vi "Dashboard Main.vi"() -> ()   [LabVIEW 2011]
uses:
  <vilib>/Rock Robotics/WPI/DriverStation/WPI_DriverStationDigitalData.ctl
panel:
  out "8 -- Battery":sgl(graph)
  out "Analog Input":sgl[](array[slide]) scale=0.0..5.0
  in  "Viewer":enum32{"Camera Image", "Kinect Skeleton"}(tab)
  in  "Video Enable":bool=TRUE
  out "Camera Image":T1(plugin-control)
  out "Buttons 1":cluster{"1":bool, "2":bool, "3":bool}
  out "Kinect 1":cluster{"X":dbl, "Y":dbl, "Z":dbl} {"X" scale=1.0..-1.0; "Y" scale=1.0..-1.0; "Z" scale=1.0..-1.0}
  out "Buttons 2":cluster{"1":bool, "2":bool, "3":bool}
  out "Kinect 2":cluster{"X":dbl, "Y":dbl, "Z":dbl} {"X" scale=1.0..-1.0; "Y" scale=1.0..-1.0; "Z" scale=1.0..-1.0}
  out "Version":string
  out "Skeleton Picture":picture
  out "Players":i8
  out "Dashboard Datatype Warning":string="Warning: The Dashboard Datatype used by the robot project and this dashboard do not match.\nSee diagram for more details."
  out "Robot IP Address":string
  out "Image Error Message":string="Timeout in Camera Communications"
  out "Solenoid Output":bool[](array[boolean])
  out "PWM":cluster{u8, u8}[](array[slide])=[{0, 157}, {0, 157}, {0, 157}, {0, 157}, {0, 157}, {0, 157}, {0, 157}, {0, 157}, {0, 157}, {0, 169}] scale=1.0..255.0
  out "GPIO Output Enable":bool[](array[boolean])
  out "GPIO State":bool[](array[boolean])
  out "Relay":cluster{"Forward":bool[], "Reverse":bool[]}
  # "Analog #1"
  # "1"
  # "7"
  # "Communications"
  # "Solenoid #1"
  # "1"
  # "8"
  # "Digital #1"
  # "1"
  # "10"
  # "1"
  # "14"
  # "1"
  # "8"
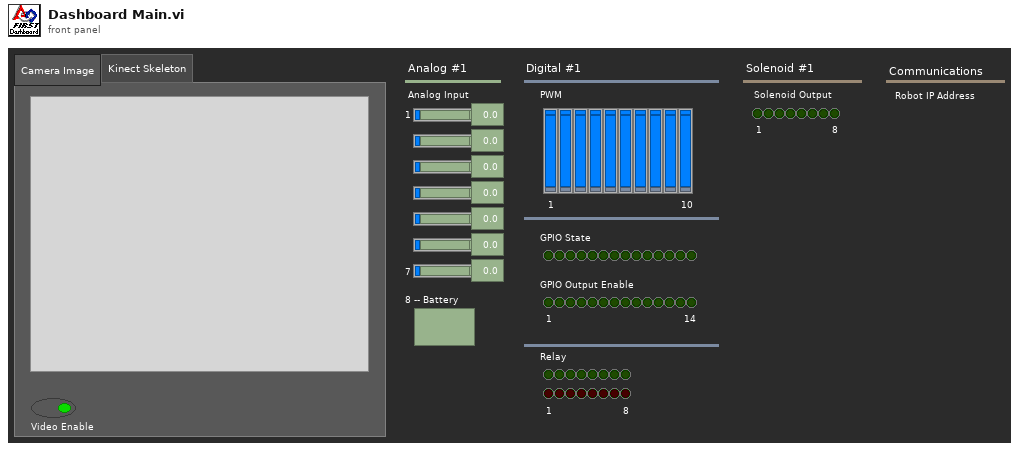
[diagram p1: front panel]
types:
  T1 = typedef "IMAQ Image.ctl" = refnum<image>
  T2 = typedef "WPI_DriverStationDigitalData.ctl" = cluster{"Relay Fwd":u8, "Relay Rev":u8, "GPIO":u16, "GPIO_OE":u16, "PWM":cluster{"PWM[0]":u8, "PWM[1]":u8, "PWM[2]":u8, "PWM[3]":u8, "PWM[4]":u8, "PWM[5]":u8, "PWM[6]":u8, "PWM[7]":u8, "PWM[8]":u8, "PWM[9]":u8}}
  T3 = cluster{cluster{"AnalogModule[0]":cluster{"Channel[0]":sgl, "Channel[1]":sgl, "Channel[2]":sgl, "Channel[3]":sgl, "Channel[4]":sgl, "Channel[5]":sgl, "Channel[6]":sgl, "Channel[7]":sgl}, "AnalogModule[1]":cluster{"Channel[0]":sgl, "Channel[1]":sgl, "Channel[2]":sgl, "Channel[3]":sgl, "Channel[4]":sgl, "Channel[5]":sgl, "Channel[6]":sgl, "Channel[7]":sgl}}, cluster{"DigitalModule[0]":T2, "DigitalModule[1]":T2}, "Solenoid":u8}
  T4 = typedef "Image Type" = u32
  T5 = cluster{"Competition mode":bool, "Robot Link":bool, "Autonomous":bool, "Enabled":bool, "E-Stop":bool}
  T6 = cluster{"AnalogModule[0]":cluster{"Channel[0]":sgl, "Channel[1]":sgl, "Channel[2]":sgl, "Channel[3]":sgl, "Channel[4]":sgl, "Channel[5]":sgl, "Channel[6]":sgl, "Channel[7]":sgl}, "AnalogModule[1]":cluster{"Channel[0]":sgl, "Channel[1]":sgl, "Channel[2]":sgl, "Channel[3]":sgl, "Channel[4]":sgl, "Channel[5]":sgl, "Channel[6]":sgl, "Channel[7]":sgl}}
  T7 = cluster{"DigitalModule[0]":T2, "DigitalModule[1]":T2}
  T8 = cluster{"Channel[0]":sgl, "Channel[1]":sgl, "Channel[2]":sgl, "Channel[3]":sgl, "Channel[4]":sgl, "Channel[5]":sgl, "Channel[6]":sgl, "Channel[7]":sgl}[]
  T9 = cluster{"Channel[0]":sgl, "Channel[1]":sgl, "Channel[2]":sgl, "Channel[3]":sgl, "Channel[4]":sgl, "Channel[5]":sgl, "Channel[6]":sgl, "Channel[7]":sgl}
  T10 = typedef "LVRectTypeDef.ctl" = cluster{"left":i16, "top":i16, "right":i16, "bottom":i16}
  T11 = typedef "SkeletonTrackState.ctl" = enum32{"NotTracked", "PositionOnly", "Tracked"}
  T12 = cluster{"TrackingState":u8[], "Position":cluster{"x":sgl, "y":sgl, "z":sgl}, cluster{"x":sgl, "y":sgl, "z":sgl, sgl}[], "TrackState":T11}
  T13 = cluster{cluster{"ScaledToPercentRange":dbl, "ScaledToPercentRange":dbl, "ScaledToPercentRange":dbl}, cluster{bool, bool, bool}}[]
  T14 = typedef "LVBoundsTypeDef.ctl" = cluster{"Width":u32, "Height":u32}
  T15 = cluster{cluster{"ScaledToPercentRange":dbl, "ScaledToPercentRange":dbl, "ScaledToPercentRange":dbl}, cluster{bool, bool, bool}}
  T16 = cluster{"ScaledToPercentRange":dbl, "ScaledToPercentRange":dbl, "ScaledToPercentRange":dbl}
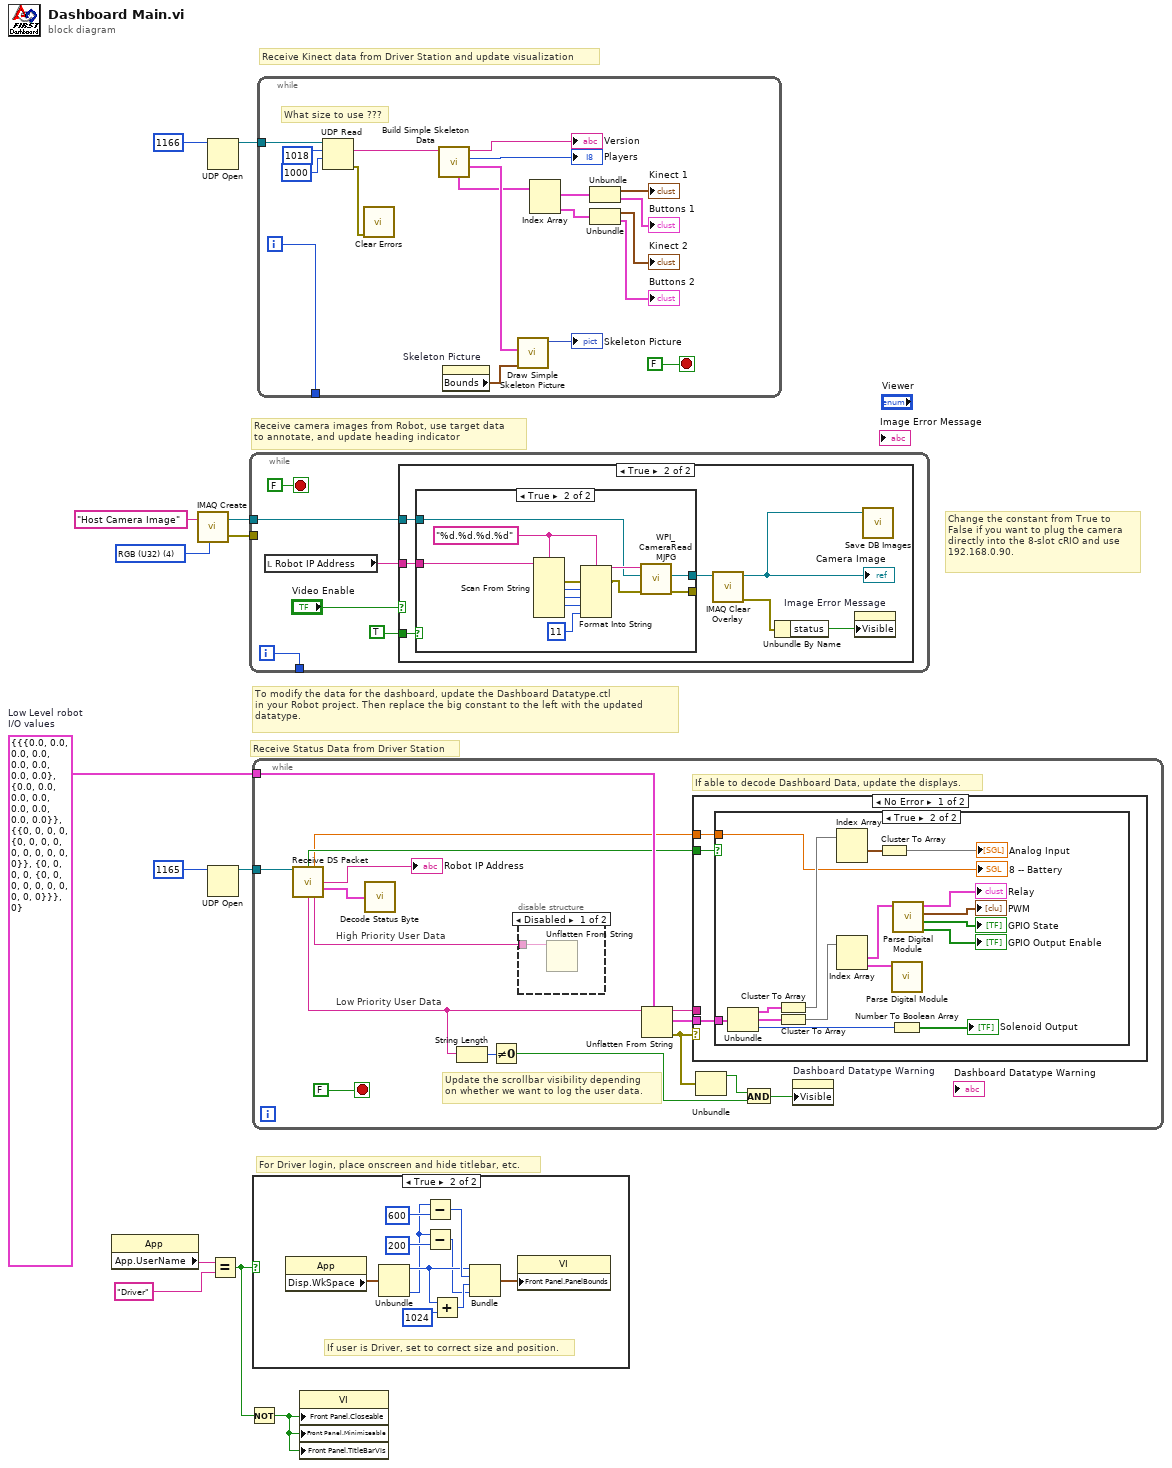
[diagram p0: block diagram]
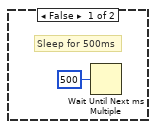
[diagram p6: hidden frame]
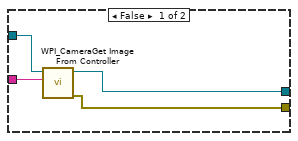
[diagram p7: hidden frame]
diagram:
  w3 = T3 {{"AnalogModule[0]"={"Channel[0]"=0.0, "Channel[1]"=0.0, "Channel[2]"=0.0, "Channel[3]"=0.0, "Channel[4]"=0.0, "Channel[5]"=0.0, "Channel[6]"=0.0, "Channel[7]"=0.0}, "AnalogModule[1]"={"Channel[0]"=0.0, "Channel[1]"=0.0, "Channel[2]"=0.0, "Channel[3]"=0.0, "Channel[4]"=0.0, "Channel[5]"=0.0, "Channel[6]"=0.0, "Channel[7]"=0.0}}, {"DigitalModule[0]"={"Relay Fwd"=0, "Relay Rev"=0, "GPIO"=0, "GPIO_OE"=0, "PWM"={"PWM[0]"=0, "PWM[1]"=0, "PWM[2]"=0, "PWM[3]"=0, "PWM[4]"=0, "PWM[5]"=0, "PWM[6]"=0, "PWM[7]"=0, "PWM[8]"=0, "PWM[9]"=0}}, "DigitalModule[1]"={"Relay Fwd"=0, "Relay Rev"=0, "GPIO"=0, "GPIO_OE"=0, "PWM"={"PWM[0]"=0, "PWM[1]"=0, "PWM[2]"=0, "PWM[3]"=0, "PWM[4]"=0, "PWM[5]"=0, "PWM[6]"=0, "PWM[7]"=0, "PWM[8]"=0, "PWM[9]"=0}}}, "Solenoid"=0}  # Low Level robot I/O values
  w11 = T4 4 items=["Grayscale (U8)", "Grayscale (I16)", "Grayscale (SGL)", "Complex (CSG)", "RGB (U32)", "HSL (U32)", "RGB (U64)"] ("Image Type")
  # "Change the constant from True to\nFalse if you want to plug the camera\ndirectly into the 8-slot cRIO and use\n192.168.0.90."
  # "Receive Kinect data from Driver Station and update visualization"
  # "For Driver login, place onscreen and hide titlebar, etc."
  # "To modify the data for the dashboard, update the Dashboard Datatype.ctl\nin your Robot project. Then replace the big constant to the left with the updated\ndatatype."
  # "Receive Status Data from Driver Station"
  # "Receive camera images from Robot, use target data\nto annotate, and update heading indicator"
  n1 = property class="App"() -> ("App.UserName"=w6:string)  [unwired: 2 in, 2 out]
  n2 = call "IMAQ Create"("Image Name"="Host Camera Image", "Image Type"=w11) -> ("New Image"=w9:T1, "error out"=w8:errorcluster)  [unwired: 2 in, 1 out]
  n3 = UDP Open(11:u16 1166 ("port")) -> (port=w1:refnum<k16>)  [unwired: 2 in, 4 out]
  n4 = UDP Open(11:u16 1165 ("port")) -> (port=w12:refnum<k16>)  [unwired: 2 in, 4 out]
  n5 = Equal?(x=w6, y="Driver") -> (x = y?=w5:bool)
  n6 = Not(x=w5) -> (.not. x?=w4:bool)
  n7 = while {
    tunnel: w9 -> [w17]
    tunnel: w8 -> [_]
    tunnel: [w14] -> _
    i -> [w14]
    stop <- FALSE stop-if-true
    n8 = local read "Robot IP Address"() -> (w18:string)
    n9 = case shown="True" "Video Enable" {
      tunnel: w18 -> [_ w27]
      tunnel: w17 -> [_ w26]
      tunnel: TRUE -> [_ w21]
      frame False {
        # "Sleep for 500ms"
        n10 = Wait Until Next ms Multiple(millisecond multiple=u32 500) -> ()  [unwired: 1 out]
      }
      frame True {
        n11 = case shown="True" w21 {
          tunnel: w26 -> [w30 w37]
          tunnel: [w28 w35] -> _
          tunnel: [w29 w36] -> w23
          tunnel: w27 -> [w31 w40]
          frame False {
            n12 = call <vilib>:"WPI_CameraGet Image From Controller.vi"("Controller Address"=w31, "Image"=w30) -> ("error out"=w28:errorcluster, "Image Out"=w29:T1)  [unwired: 2 in, 6 out]
          }
          frame True {
            w32 = "%d.%d.%d.%d" ("format string")
            n13 = Scan From String(format string=w32, input string=w40) -> (error out=w39:errorcluster, output 1=w41:i32, output 2=w42:i32, output 3=w43:i32)  [unwired: 2 in, 7 out]
            n14 = Format Into String(format string=w32, error in=w39, w41, w42, w43, 11 ("IP Suffix:")) -> (resulting string=w38:string, error out=w34:errorcluster)  [unwired: 1 in]
            n15 = call <vilib>:"WPI_CameraRead MJPG.vi"("error in"=w34, "Image"=w37, "address"=w38) -> ("error out"=w35:errorcluster, "Image Out"=w36:T1)  [unwired: 7 in]
          }
        }
        n16 = call "IMAQ Clear Overlay"("Image"=w23) -> ("error out"=w24:errorcluster, "Image Out"=w22:T1)  [unwired: 2 in, 7 out]
        "Camera Image" <- w22
        n17 = Unbundle By Name(w24) -> ("status"=w25:bool)
        n18 = property on="Image Error Message" class="Str"("Visible"=w25) -> ()  [unwired: 2 in, 2 out]
        n19 = call "Save DB Images.vi"("Image"=w22) -> ()  [unwired: 2 in, 1 out]
      }
    }
  }
  n20 = while {
    tunnel: w12 -> [w57]
    tunnel: w3 -> [w56]
    stop <- FALSE stop-if-true
    # "High Priority User Data"
    # "Low Priority User Data"
    # "Update the scrollbar visibility depending\non whether we want to log the user data."
    # "If able to decode Dashboard Data, update the displays."
    n21 = call "Receive DS Packet.vi"("Recv Socket"=w57) -> ("New Dashboard Data"=w53:bool, "Battery"=w44:sgl, "Robot IP Address"=→"Robot IP Address":string, "Status"=w58:T5, "Low Priority User Data"=w46:string, "High Priority User Data"=w45:string)  [unwired: 1 in, 8 out]
    n22 = call "Decode Status Byte.vi"("Status Byte"=w58) -> ()  [unwired: 2 out]
    n23 = String Length(string=w46) -> (length=w48:i32)
    n24 = Not Equal To 0?(x=w48) -> (x != 0?=w51:bool)
    n25 = disable-structure shown="Disabled" {
      disable-tunnel: w45 -> [w60 _]
      frame Disabled {
        n26 = Unflatten From String(binary string=w60) -> ()  [unwired: 2 in, 5 out]
      }
      frame Enabled {
      }
    }
    n27 = Unflatten From String(type=w56, binary string=w46) -> (rest of the binary string=w49:string, value=w55:T3, error out=w54:errorcluster)  [unwired: 1 in, 2 out]
    n28 = case shown="No Error" w54 {
      tunnel: w55 -> [w63 _]
      tunnel: w53 -> [w62 _]
      tunnel: w49 -> [_ _]
      tunnel: w44 -> [w61 _]
      frame No Error {
        n29 = case shown="True" w62 {
          tunnel: w63 -> [_ w70]
          tunnel: w61 -> [_ w64]
          frame False {
            # "Don't update if the robot hasn't sent new data"
          }
          frame True {
            n30 = Unbundle(w70) -> (w67:T6, w68:T7, "Solenoid"=w69:u8)
            n31 = Cluster To Array(cluster=w67) -> (array=w78:T8)
            n32 = Cluster To Array(cluster=w68) -> (array=w77:T2[])
            n33 = Index Array(array=w78) -> (element #1=w65:T9)  [unwired: 2 in, 1 out]
            n34 = Index Array(array=w77) -> (element #1=w76:T2, element #2=w71:T2)  [unwired: 2 in]
            n35 = Cluster To Array(cluster=w65) -> (array=→"Analog Input":sgl[])
            n36 = call "Parse Digital Module.vi"("DigitalModule"=w71) -> ()  [unwired: 11 out]
            n37 = Number To Boolean Array(number=w69) -> (Boolean array=→"Solenoid Output":bool[])
            n38 = call "Parse Digital Module.vi"("DigitalModule"=w76) -> ("GPIO Output Enable"=→"GPIO Output Enable":bool[], "GPIO State"=→"GPIO State":bool[], "PWM"=→"PWM":cluster{u8, u8}[], "Relay"=→"Relay":cluster{"Forward":bool[], "Reverse":bool[]})  [unwired: 7 out]
            "8 -- Battery" <- w64
          }
        }
      }
      frame Error {
        # "Your datatypes don't match. The Dashboard Datatype.ctl in your Robot project\nand the big constant to the left of the loop need to match."
      }
    }
    n39 = Unbundle(w54) -> ("status"=w50:bool)  [unwired: 2 out]
    n40 = And(x=w50, y=w51) -> (x .and. y?=w52:bool)
    n41 = property on="Dashboard Datatype Warning" class="Str"("Visible"=w52) -> ()  [unwired: 2 in, 2 out]
  }
  n42 = case shown="True" w5 {
    frame False {
    }
    frame True {
      # "If user is Driver, set to correct size and position."
      n43 = property class="App"() -> ("Disp.WkSpace"=w89:T10)  [unwired: 2 in, 2 out]
      n44 = Unbundle(w89) -> ("left"=w84:i16, "bottom"=w80:i16)  [unwired: 2 out]
      n45 = Subtract(x=w80, y=600) -> (x-y=w86:i32)
      n46 = Subtract(x=w80, y=200) -> (x-y=w81:i32)
      n47 = Add(x=w84, y=1024) -> (x+y=w85:i32)
      n48 = Bundle("left"=w84, w86, w85, w81) -> (w88:cluster{"left":i16, i32, i32, i32})  [unwired: 1 out]
      n49 = property class="VI"("Front Panel.PanelBounds"=w88) -> ()  [unwired: 2 in, 2 out]
    }
  }
  n50 = while {
    tunnel: w1 -> [w106]
    tunnel: [w90] -> _
    i -> [w90]
    stop <- FALSE stop-if-true
    # "What size to use ???"
    n51 = UDP Read(connection ID=w106, max size (548)=1018 ("bytes to read"), timeout ms (25000)=1000) -> (data out=w100:string, error out=w98:errorcluster)  [unwired: 1 in, 3 out]
    n52 = call <vilib>:"Clear Errors.vi"("error in (no error)"=w98) -> ()  [unwired: 6 in, 1 out]
    n53 = call "Build Simple Skeleton Data.vi"("data out"=w100) -> ("Skeleton Data"=w101:T12, "NumPlayers"=→"Players":i8, "Version String"=→"Version":string, "Simple Joystick Info"=w97:T13)  [unwired: 6 in, 1 out]
    n54 = property on="Skeleton Picture" class="Pict"() -> ("Bounds"=w102:T14)  [unwired: 2 in, 2 out]
    n55 = call "Draw Simple Skeleton Picture.vi"("Bounds"=w102, "Simple Skeleton"=w101) -> ("new picture out"=→"Skeleton Picture":picture)  [unwired: 9 in]
    n56 = Index Array(array=w97) -> (element #1=w96:T15, element #2=w95:T15)  [unwired: 2 in]
    n57 = Unbundle(w96) -> (→"Kinect 1":T16, →"Buttons 1":cluster{bool, bool, bool})
    n58 = Unbundle(w95) -> (→"Kinect 2":T16, →"Buttons 2":cluster{bool, bool, bool})
  }
  n59 = property class="VI"("Front Panel.Closeable"=w4, "Front Panel.Minimizeable"=w4, "Front Panel.TitleBarVis"=w4) -> ()  [unwired: 2 in, 2 out]
